vi "Untitled 6.vi"(0 "input cluster":T2) -> (1 "Strafe":dbl, 2 "Forward/Reverse":dbl, 3 "Turn":dbl)   [LabVIEW 2013]
uses:
  <vilib>/Rock Robotics/WPI/Joystick/WPI_JoystickButtonState.ctl
panel:
  out "Picker Upper":bool
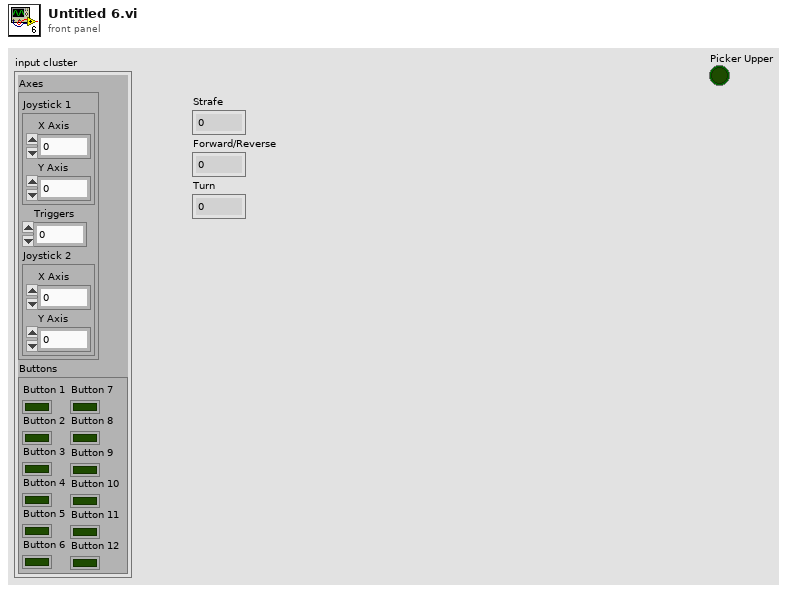
[diagram p1: front panel]
types:
  T1 = typedef "WPI_JoystickButtonState.ctl" = cluster{"Button 1":bool, "Button 2":bool, "Button 3":bool, "Button 4":bool, "Button 5":bool, "Button 6":bool, "Button 7":bool, "Button 8":bool, "Button 9":bool, "Button 10":bool, "Button 11":bool, "Button 12":bool}
  T2 = cluster{"Axes":cluster{"Joystick 1":cluster{"X Axis":dbl, "Y Axis":dbl}, "Triggers":dbl, "Joystick 2":cluster{"X Axis":dbl, "Y Axis":dbl}}, "Buttons":T1}
  T3 = cluster{"Joystick 1":cluster{"X Axis":dbl, "Y Axis":dbl}, "Triggers":dbl, "Joystick 2":cluster{"X Axis":dbl, "Y Axis":dbl}}
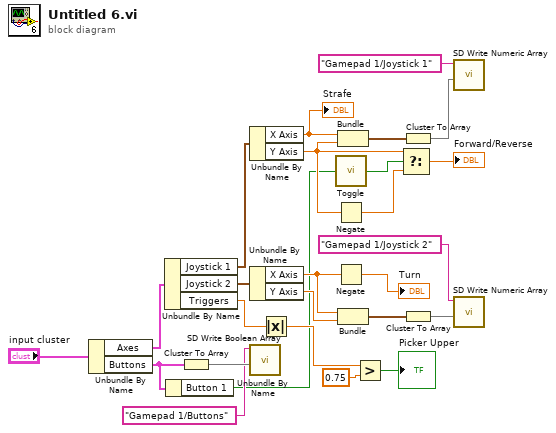
[diagram p0: block diagram]
diagram:
  n1 = Unbundle By Name("input cluster") -> ("Axes"=w26:T3, "Buttons"=w3:T1)
  n2 = Unbundle By Name(w26) -> ("Joystick 1"=w25:cluster{"X Axis":dbl, "Y Axis":dbl}, "Joystick 2"=w16:cluster{"X Axis":dbl, "Y Axis":dbl}, "Triggers"=w11:dbl)
  n3 = Unbundle By Name(w3) -> ("Button 1"=w2:bool)
  n4 = Cluster To Array(cluster=w3) -> (array=w5:bool[])
  n5 = Unbundle By Name(w25) -> ("X Axis"=w24:dbl, "Y Axis"=w13:dbl)
  "Strafe" <- w24
  n6 = Unbundle By Name(w16) -> ("X Axis"=w17:dbl, "Y Axis"=w19:dbl)
  n7 = call <vilib>:"SD Write Boolean Array.vi"("Boolean Array"=w5, "Name"="Gamepad 1/Buttons") -> ()  [unwired: 8 in, 2 out]
  n8 = Absolute Value(x=w11) -> (abs(x)=w10:dbl)
  n9 = call "Toggle.vi"("Input"=w2) -> ("Latched"=w8:bool)
  n10 = Negate(x=w13) -> (-x=w12:dbl)
  n11 = Negate(x=w17) -> (-x=→"Turn":dbl)
  n12 = Bundle("X Axis"=w24, "Y Axis"=w13) -> (w14:cluster{"X Axis":dbl, "Y Axis":dbl})  [unwired: 1 in]
  n13 = Bundle("X Axis"=w17, "Y Axis"=w19) -> (w21:cluster{"X Axis":dbl, "Y Axis":dbl})  [unwired: 1 in]
  n14 = Greater?(x=w10, y=0.75) -> (0:→"Picker Upper":bool)
  n15 = Select(t=w13, s=w8, f=w12) -> (s? t:f=→"Forward/Reverse":dbl)
  n16 = Cluster To Array(cluster=w14) -> (array=w23:dbl[])
  n17 = Cluster To Array(cluster=w21) -> (array=w20:dbl[])
  n18 = call <vilib>:"SD Write Numeric Array.vi"("Numeric Array"=w23, "Name"="Gamepad 1/Joystick 1") -> ()  [unwired: 8 in, 2 out]
  n19 = call <vilib>:"SD Write Numeric Array.vi"("Numeric Array"=w20, "Name"="Gamepad 1/Joystick 2") -> ()  [unwired: 8 in, 2 out]
